vi "8xU8 to U64.vi"(1 "8xU8":u8[](array[numeric])=[0, 0, 0, 0, 0, 0, 0, 0] format="%x") -> (0 "U64":u64)   [LabVIEW 2016]
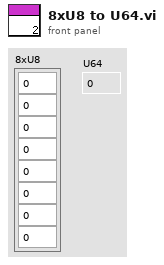
[diagram p1: front panel]
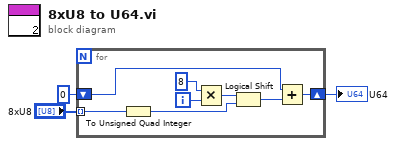
[diagram p0: block diagram]
diagram:
  n1 = for {
    shift-right: [w5] -> w1
    shift-left: u64 0 -> [w7]
    tunnel: "8xU8" -> [w4] mode=indexing
    i -> [w9]
    n2 = To Unsigned Quad Integer(1:w4) -> (0:w6:u64)
    n3 = Multiply(x=i8 8, y=w9) -> (x*y=w8:i32)
    n4 = Logical Shift(y=w8, x=w6) -> (x << y=w11:u64)
    n5 = Add(x=w7, y=w11) -> (x+y=w5:u64)
  }
  "U64" <- w1
